vi "optionsAcq_rangeCheck.vi"(0 "range min (waveNr)":sgl, 1 "channel index spectrum":u16, 2 "spectrometerIdx":u16, 3 "update mode":enum16{"range min", "range max", "both"}(ring), 5 "range max (waveNr)":sgl, 7 "range current min":sgl, 9 "range current max":sgl, 11 "error in":errorcluster, 12 "waveNrMin support":sgl, 13 "waveNrMax support":sgl) -> (4 "range min (waveNr) out":sgl, 6 "range max (waveNr) out":sgl, 15 "error out":errorcluster)   [LabVIEW 2010, in "OSA.lvclass"]
uses:
  OSA.lvclass
  OSA20X_misc.lvlib
  FTSLib.dll
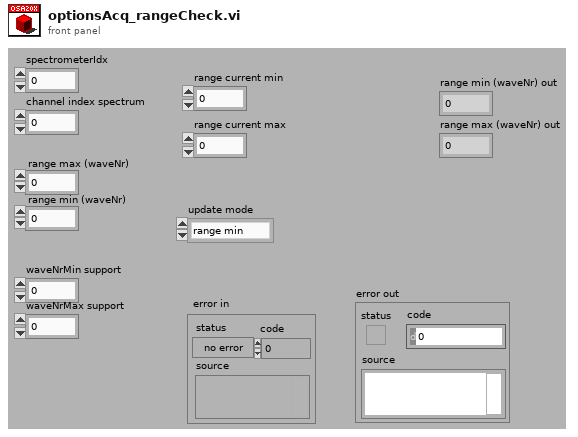
[diagram p1: front panel]
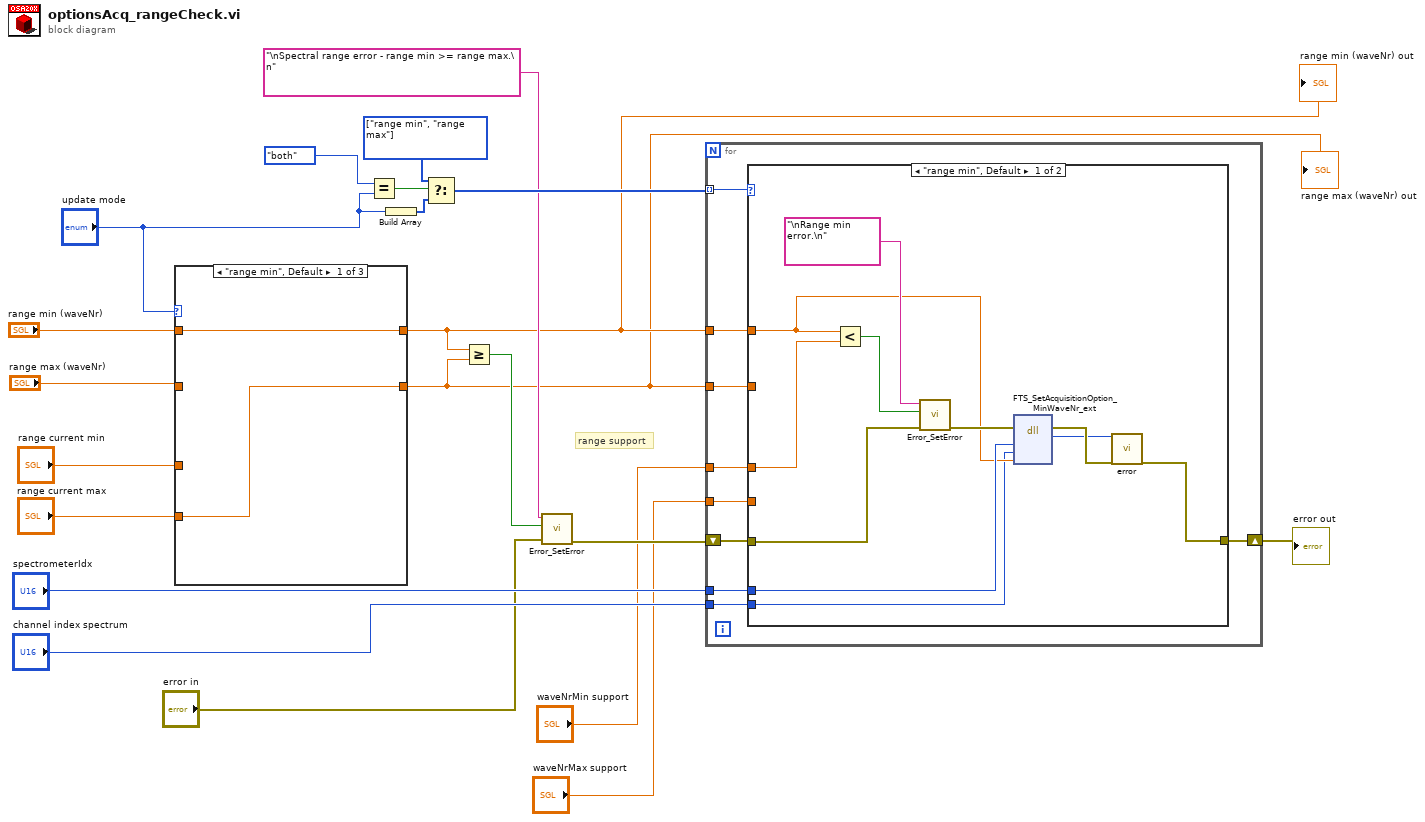
[diagram p0: block diagram]
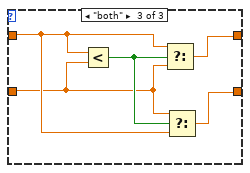
[diagram p3: hidden frame]
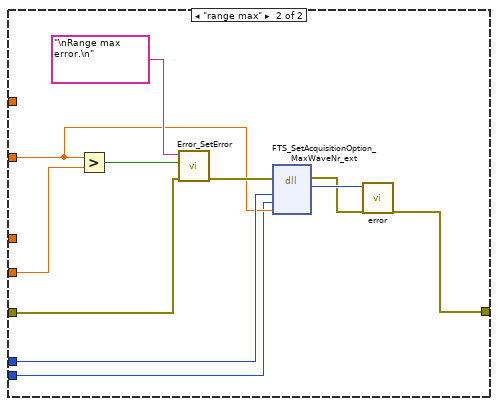
[diagram p4: hidden frame]
diagram:
  w19 = enum16{"range min", "range max", "both"}[] [enum."range min", enum."range max"] items=["range min", "range max", "both"]
  # "range support"
  n1 = case shown="\"range min\", Default" "update mode" {
    tunnel: "range max (waveNr)" -> [_ w25 w28]
    tunnel: [w22 w25 w26] -> w12
    tunnel: [w23 w24 w27] -> w13
    tunnel: "range current min" -> [_ w24 _]
    tunnel: "range min (waveNr)" -> [w23 _ w29]
    tunnel: "range current max" -> [w22 _ _]
    frame "range min", Default {
    }
    frame "range max" {
    }
    frame "both" {
      n2 = Less?(x=w29, y=w28) -> (x < y?=w30:bool)
      n3 = Select(t=w29, s=w30, f=w28) -> (s? t:f=w27:sgl)
      n4 = Select(t=w28, s=w30, f=w29) -> (s? t:f=w26:sgl)
    }
  }
  "range min (waveNr) out" <- w13
  "range max (waveNr) out" <- w12
  n5 = Equal?(x=enum16{"range min", "range max", "both"}."both" ("action"), y="update mode") -> (x = y?=w20:bool)
  n6 = Build Array("update mode") -> (w18:enum16{"range min", "range max", "both"}[])
  n7 = Select(t=w19, s=w20, f=w18) -> (s? t:f=w17:enum16{"range min", "range max", "both"}[])
  n8 = Greater Or Equal?(x=w13, y=w12) -> (x >= y?=w16:bool)
  n9 = call "Error_SetError.vi"("error in"="error in", "status (true)"=w16, "source(\"\")"="\nSpectral range error - range min >= range max.\n" ("source(\"\")")) -> ("error out"=w11:errorcluster)  [unwired: 4 in]
  n10 = for {
    tunnel: "waveNrMin support" -> [w39]
    tunnel: "waveNrMax support" -> [w38]
    tunnel: w13 -> [w37]
    tunnel: w12 -> [w36]
    tunnel: w17 -> [w35] mode=indexing
    tunnel: "spectrometerIdx" -> [w34]
    shift-right: [w32] -> w14
    shift-left: w11 -> [w33]
    tunnel: "channel index spectrum" -> [w31]
    n11 = case shown="\"range min\", Default" w35 {
      tunnel: w33 -> [w49 w58]
      tunnel: w39 -> [w50 _]
      tunnel: w38 -> [_ w59]
      tunnel: w37 -> [w44 _]
      tunnel: w36 -> [_ w52]
      tunnel: w34 -> [w46 w56]
      tunnel: [w42 w53] -> w32
      tunnel: w31 -> [w40 w51]
      frame "range min", Default {
        n12 = Less?(x=w44, y=w50) -> (x < y?=w48:bool)
        n13 = call "Error_SetError.vi"("error in"=w49, "status (true)"=w48, "source(\"\")"="\nRange min error.\n" ("source(\"\")")) -> ("error out"=w45:errorcluster)  [unwired: 4 in]
        n14 = dll-call lib="FTSLib.dll" fn="FTS_SetAcquisitionOption_MinWaveNr_ext" label="FTS_SetAcquisitionOption_MinWaveNr"(error in=w45, "spectrIdx"=w46, "channel"=w40, "waveNr_min"=w44) -> (error out=w43:errorcluster, "return type"=w41:i32)  [unwired: 5 in, 1 out]
        n15 = call "error.vi"("result code"=w41, "error in (no error)"=w43) -> ("error out"=w42:errorcluster)  [unwired: 15 in, 2 out]
      }
      frame "range max" {
        n16 = Greater?(x=w52, y=w59) -> (0:w57:bool)
        n17 = call "Error_SetError.vi"("error in"=w58, "status (true)"=w57, "source(\"\")"="\nRange max error.\n" ("source(\"\")")) -> ("error out"=w60:errorcluster)  [unwired: 4 in]
        n18 = dll-call lib="FTSLib.dll" fn="FTS_SetAcquisitionOption_MaxWaveNr_ext" label="FTS_SetAcquisitionOption_MaxWaveNr"(error in=w60, "spectrIdx"=w56, "channel"=w51, "waveNr_min"=w52) -> (error out=w54:errorcluster, "return type"=w55:i32)  [unwired: 5 in, 1 out]
        n19 = call "error.vi"("result code"=w55, "error in (no error)"=w54) -> ("error out"=w53:errorcluster)  [unwired: 15 in, 2 out]
      }
    }
  }
  "error out" <- w14
